vi "Set Min Size to Current.vi"(8 "error in (no error)":errorcluster, 11 "Pane in":refnum<class "Pane.lvclass">) -> (0 "error out":errorcluster, 2 "Min Pane Size":T1, 3 "Pane out":refnum<class "Pane.lvclass">)   [LabVIEW 2015, in "Pane.lvclass"]
uses:
  Pane.lvclass
  <vilib>/Utility/miscctls.llb/LVPointTypeDef.ctl
  Pane.lvclass/Pane.ctl
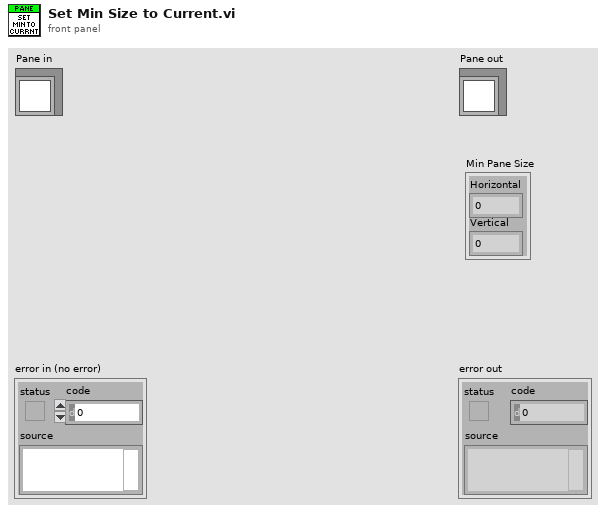
[diagram p1: front panel]
types:
  T1 = typedef "LVPointTypeDef.ctl" = cluster{"Horizontal":i16, "Vertical":i16}
  T2 = typedef "LVRectTypeDef.ctl" = cluster{"Left":i16, "Top":i16, "Right":i16, "Bottom":i16}
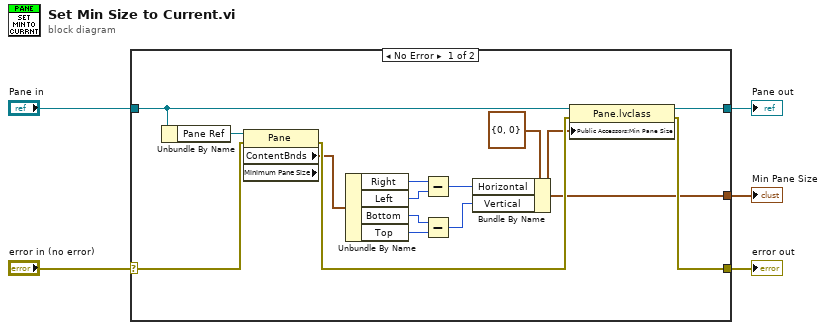
[diagram p0: block diagram]
diagram:
  n1 = case shown="No Error" "error in (no error)" {
    selector: "error in (no error)" -> [w19 w22]
    tunnel: [w9 w22] -> w4
    tunnel: [w13 w21] -> w2
    tunnel: "Pane in" -> [w14 w21]
    tunnel: [w8 _] -> w1
    frame No Error {
      n2 = Unbundle By Name(w14) -> ("Pane Ref"=w20:refnum<vi>)
      n3 = property class="Pane" props=["ContentBnds", "Minimum Pane Size"](reference=w20, error in=w19) -> (error out=w10:errorcluster, "ContentBnds"=w7:T2)  [unwired: 2 out]
      n4 = Unbundle By Name(w7) -> ("Right"=w18:i16, "Left"=w17:i16, "Bottom"=w15:i16, "Top"=w16:i16)
      n5 = Subtract(x=w18, y=w17) -> (x-y=w12:i16)
      n6 = Subtract(x=w15, y=w16) -> (x-y=w11:i16)
      n7 = Bundle By Name(cluster=T1 {"Horizontal"=0, "Vertical"=0} ("Minimum Pane Size"), "Horizontal"=w12, "Vertical"=w11) -> (w8:T1)
      n8 = property class="Pane.lvclass"(reference=w14, error in=w10, "Public Accessors:Min Pane Size"=w8) -> (reference out=w13:refnum<class "Pane.lvclass">, error out=w9:errorcluster)
    }
    frame Error {
    }
  }
  "error out" <- w4
  "Pane out" <- w2
  "Min Pane Size" <- w1
